vi "createNode.vi"(8 "error in (no error)":errorcluster, 10 "NodeSelection":T1, 11 "NodeFactory in":refnum<class "NodeFactory.lvclass">) -> (0 "error out":errorcluster, 2 "Node":refnum<class "Node.lvclass">, 3 "NodeFactory out":refnum<class "NodeFactory.lvclass">)   [LabVIEW 2016, in "NodeFactory.lvclass"]
uses:
  NodeFactory.lvclass
  Node/Node.lvclass
  Typedefs/NodeSelection.ctl
  Nodes/DefaultNode/DefaultNode.lvclass
  C:/LSST_TS/SystemSW/ct_tools/Node/Node.lvclass
  Nodes/CaseStructure/CaseStructure.lvclass
  Nodes/EventStructure/EventStructure.lvclass
  Nodes/FlatSequence/FlatSequence.lvclass
  Nodes/ForLoop/ForLoop.lvclass
  Nodes/WhileLoop/WhileLoop.lvclass
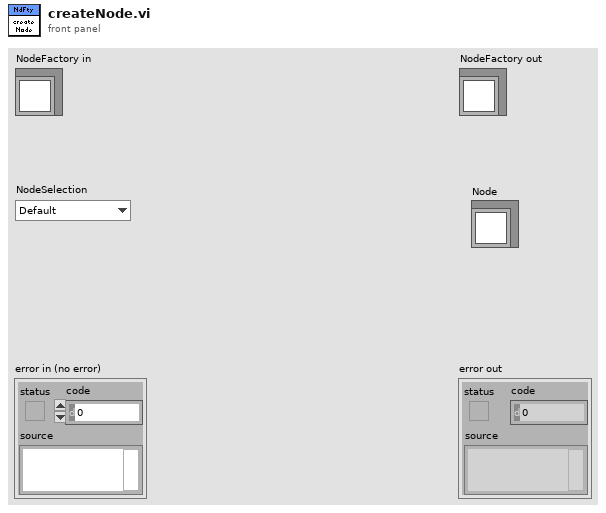
[diagram p1: front panel]
types:
  T1 = typedef "NodeSelection.ctl" = enum16{"Default", "CaseStructure", "EventStructure", "FlatSequence", "ForLoop", "WhileLoop"}
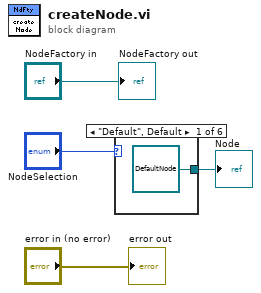
[diagram p0: block diagram]
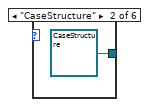
[diagram p2: hidden frame]
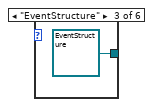
[diagram p3: hidden frame]
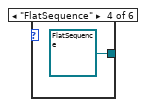
[diagram p4: hidden frame]
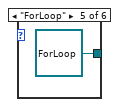
[diagram p5: hidden frame]
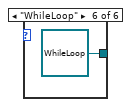
[diagram p6: hidden frame]
diagram:
  n1 = case shown="\"Default\", Default" "NodeSelection" {
    tunnel: [refnum<class "DefaultNode.lvclass"> refnum ("DefaultNode.lvclass") refnum<class "CaseStructure.lvclass"> refnum ("CaseStructure.lvclass") refnum<class "EventStructure.lvclass"> refnum ("EventStructure.lvclass") refnum<class "FlatSequence.lvclass"> refnum ("FlatSequence.lvclass") refnum<class "ForLoop.lvclass"> refnum ("ForLoop.lvclass") refnum<class "WhileLoop.lvclass"> refnum ("WhileLoop.lvclass")] -> w1
    frame "Default", Default {
    }
    frame "CaseStructure" {
    }
    frame "EventStructure" {
    }
    frame "FlatSequence" {
    }
    frame "ForLoop" {
    }
    frame "WhileLoop" {
    }
  }
  "Node" <- w1
  "error out" <- "error in (no error)"
  "NodeFactory out" <- "NodeFactory in"
